vi "Release Semaphore.vi"(8 "error in (no error)":errorcluster, 10 "VI in":refnum<vi>, 11 "Slave Test Runner in":refnum<class "Slave Test Runner.lvclass">) -> (0 "error out":errorcluster, 2 "VI out":refnum<vi>, 3 "Slave Test Runner out":refnum<class "Slave Test Runner.lvclass">)   [LabVIEW 2020, in "Slave Test Runner.lvclass"]
uses:
  Slave Test Runner.lvclass
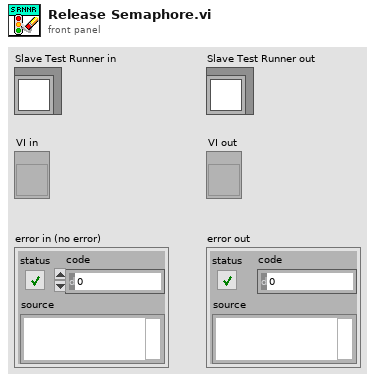
[diagram p1: front panel]
types:
  T1 = typedef "Semaphore RefNum" = refnum<k1>
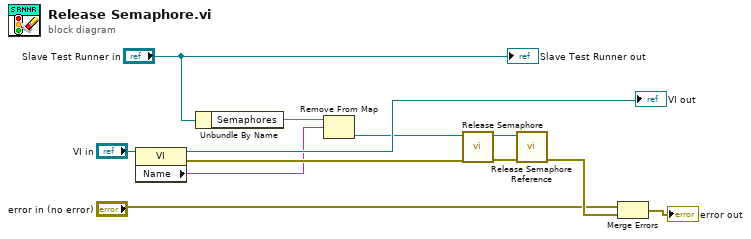
[diagram p0: block diagram]
diagram:
  n1 = property class="VI"(reference="VI in") -> (reference out=→"VI out":refnum<vi>, error out=w7:errorcluster, "Name"=w2:string)  [unwired: 1 in]
  n2 = Unbundle By Name("Slave Test Runner in") -> ("Semaphores"=w3:map{string, T1})
  n3 = Remove From Map(10:w2, 11:w3) -> (1:w1:T1)  [unwired: 2 out]
  n4 = call <vilib>:"Release Semaphore.vi"("error in (no error)"=w7, "semaphore"=w1) -> ("error out"=w11:errorcluster, "semaphore out"=w10:T1)  [unwired: 4 in]
  n5 = call <vilib>:"Release Semaphore Reference.vi"("error in (no error)"=w11, "semaphore"=w10) -> ("error out"=w12:errorcluster)  [unwired: 8 in, 1 out]
  n6 = Merge Errors("error in (no error)", w12) -> (→"error out":errorcluster)
  "Slave Test Runner out" <- "Slave Test Runner in"
